vi "Test Base Persist Arguments from Init.vi"(8 "error in (no error)":errorcluster, 11 "Base Class Test In":refnum<class "Base Dev Test.lvclass">) -> (0 "error out":errorcluster, 3 "Base Class Test Out":refnum<class "Base Dev Test.lvclass">)   [LabVIEW 2020, in "Base Dev Test.lvclass"]
uses:
  Base Dev Test.lvclass
  C:/Program Files (x86)/National Instruments/LabVIEW 2020/vi.lib/Astemes/LUnit/Test Case.lvclass
  Base Dev Test.lvclass/Base Dev Test.ctl
  source/Framework/Base/Base.lvclass/Base.ctl
  <vilib>/Astemes/LUnit/Test Case.lvclass/Test Case.ctl
  <vilib>/Astemes/LUnit/LUnit Assertion Result.lvclass/LUnit Assertion Result.ctl
  <vilib>/Astemes/LUnit/LUnit Test Case Result.lvclass/LUnit Test Case Result.ctl
  <vilib>/Astemes/LUnit/LUnit Method Result.lvclass/LUnit Method Result.ctl
  <vilib>/Astemes/LUnit/Palette/Pass If Equal.vi/cbf50e99-f124-4847-863a-8e9794d3dede.vi
  <vilib>/Astemes/LUnit/Palette/Pass.vi
  <vilib>/Astemes/LUnit/Palette/Fail.vi
  <vilib>/Astemes/LUnit/Compare Variants.vi
  <vilib>/Astemes/LUnit/Describe Comparison.vi
  <vilib>/Astemes/LUnit/Set Assertion Type.vi
  <vilib>/Astemes/LUnit/Add test result.vi
  <vilib>/Astemes/LUnit/LUnit Write Passed.vi
  <vilib>/Astemes/LUnit/LUnit Write Message.vi
  <vilib>/Astemes/LUnit/LUnit Write Description.vi
  <vilib>/Astemes/LUnit/Variant to string.vi
  <vilib>/Astemes/LUnit/LUnit Write Assertion Type.vi
  <vilib>/Astemes/LUnit/LUnit Record Assertion Result.vi
  <vilib>/Astemes/LUnit/LUnit Aggregate Assertion Results.vi
  <vilib>/Astemes/LUnit/Assertion Result/LUnit Read Status.vi
  <vilib>/Astemes/LUnit/LUnit Read Message.vi
  <vilib>/Astemes/LUnit/LUnit Read Description.vi
  <vilib>/Astemes/LUnit/Method Result/LUnit Merge Status.vi
  <vilib>/Astemes/LUnit/LUnit Concatenate result strings.vi
  <vilib>/Utility/Data Type/Get Type Information.vi
  <vilib>/Utility/LVClass/Get LV Class Name.vi
  source/Framework/Base/Base.lvclass
  <vilib>/Astemes/LUnit/LUnit Assertion Result.lvclass
  <vilib>/Astemes/LUnit/Test Case.lvclass
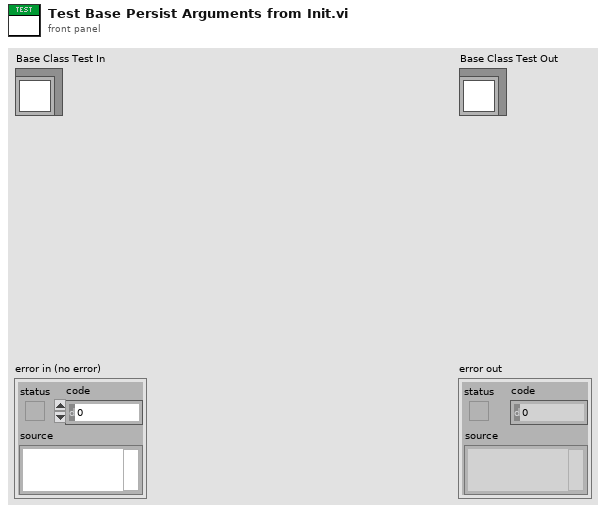
[diagram p1: front panel]
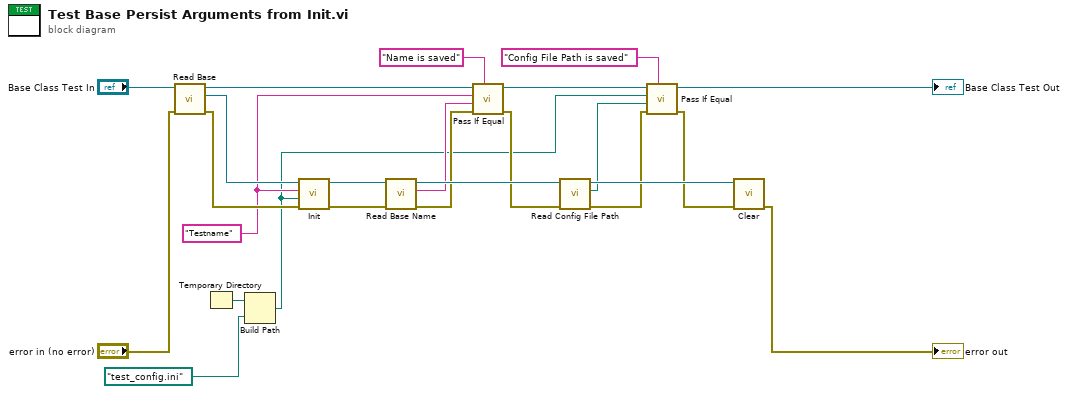
[diagram p0: block diagram]
diagram:
  w14 = "Testname" ("Name")
  n1 = call "Read Base.vi"("error in (no error)"="error in (no error)", "Base Class Test In"="Base Class Test In") -> ("error out"=w16:errorcluster, "Base.lvclass"=w18:refnum<class "Base.lvclass">, "Base Class Test Out"=w19:refnum<class "Base Dev Test.lvclass">)  [unwired: 7 in]
  n2 = Temporary Directory() -> (w3:path)
  n3 = Build Path(base path=w3, name or relative path=path "test_config.ini" ("Config File Path")) -> (appended path=w2:path)
  n4 = call-dynamic "Init.vi"("error in (no error)"=w16, "Config File Path"=w2, "Name"=w14, "Base In"=w18) -> ("error out"=w22:errorcluster, "Base Out"=w23:refnum<class "Base.lvclass">)  [unwired: 6 in]
  n5 = call "Read Base Name.vi"("error in (no error)"=w22, "Base In"=w23) -> ("error out"=w12:errorcluster, "Name"=w13:string, "Base Out"=w21:refnum<class "Base.lvclass">)  [unwired: 7 in]
  n6 = call <vilib>:"Pass If Equal.vi"("Description"="Name is saved", "error in (no error)"=w12, "Actual"=w13, "Expected"=w14, "LUnit Test Case In"=w19) -> ("error out"=w11:errorcluster, "LUnit Test Case Out"=w15:refnum<class "Base Dev Test.lvclass">)  [unwired: 5 in]
  n7 = call "Read Config File Path.vi"("error in (no error)"=w11, "Base In"=w21) -> ("error out"=w9:errorcluster, "Config File Path"=w10:path, "Base Out"=w20:refnum<class "Base.lvclass">)  [unwired: 7 in]
  n8 = call <vilib>:"Pass If Equal.vi"("Description"="Config File Path is saved", "error in (no error)"=w9, "Actual"=w10, "Expected"=w2, "LUnit Test Case In"=w15) -> ("error out"=w8:errorcluster, "LUnit Test Case Out"=→"Base Class Test Out":refnum<class "Base Dev Test.lvclass">)  [unwired: 5 in]
  n9 = call-dynamic "Clear.vi"("error in (no error)"=w8, "Base In"=w20) -> ("error out"=→"error out":errorcluster)  [unwired: 9 in]
